vi "AAL Ramp Pattern.vi"(2 "start":dbl format="%.2f", 3 "end":dbl=1.0 format="%.2f", 4 "samples":i32=128) -> (0 "error":i32, 1 "Ramp Pattern":dbl[](array[numeric]) format="%.2f")   [LabVIEW 2020, in "NI_AALPro.lvlib"]
doc: "Generates an array containing a ramp pattern."
uses:
  NI_AALPro.lvlib
  NI_AALBase.lvlib
panel:
  # "Ramp Pattern"
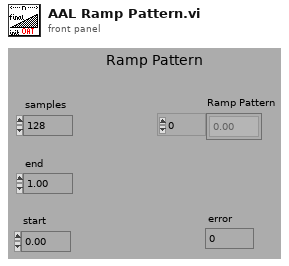
[diagram p1: front panel]
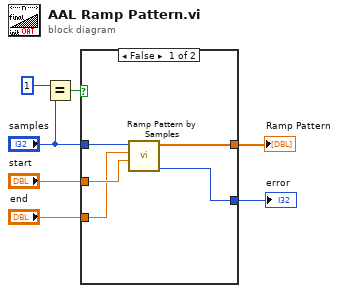
[diagram p0: block diagram]
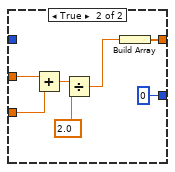
[diagram p2: hidden frame]
diagram:
  n1 = Equal?(x=1, y="samples") -> (x = y?=w1:bool)
  n2 = case shown="False" w1 {
    tunnel: "samples" -> [w12 _]
    tunnel: [w11 w15] -> w5
    tunnel: [w10 0 ("error")] -> w4
    tunnel: "start" -> [w9 w19]
    tunnel: "end" -> [w8 w18]
    frame False {
      n3 = call "Ramp Pattern by Samples.vi"("start"=w9, "end"=w8, "samples"=w12) -> ("error"=w10:i32, "Ramp Pattern"=w11:dbl[])  [unwired: 7 in]
    }
    frame True {
      n4 = Add(x=w19, y=w18) -> (x+y=w17:dbl)
      n5 = Divide(x=w17, y=2.0) -> (x/y=w14:dbl)
      n6 = Build Array(w14) -> (w15:dbl[])
    }
  }
  "Ramp Pattern" <- w5
  "error" <- w4
